vi "InitSelectRing.vi"(8 "error in (no error)":errorcluster, 11 "Ring Refnum":refnum<vi>) -> (0 "error out":errorcluster, 2 "Module Ring Value":i32=-1)   [LabVIEW 2018, in "ScopeModule.lvlib"]
uses:
  ScopeModule.lvlib
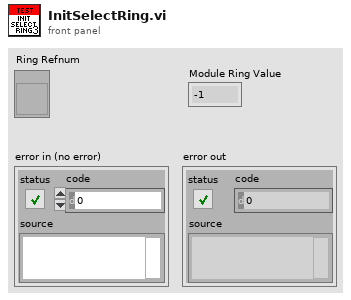
[diagram p1: front panel]
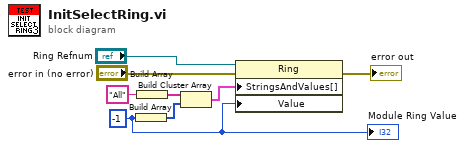
[diagram p0: block diagram]
diagram:
  w2 = -1
  n1 = Build Array(w2) -> (w6:i32[])
  n2 = Build Array("All") -> (w7:string[])
  n3 = Build Cluster Array(w7, w6) -> (w3:cluster{string, i32}[])
  n4 = property class="Ring"(reference="Ring Refnum", error in="error in (no error)", "StringsAndValues[]"=w3, "Value"=w2) -> (error out=→"error out":errorcluster)  [unwired: 1 out]
  "Module Ring Value" <- w2
